vi "Distance-Speed Adaptor.vi"(4 "Sensor Data":dbl) -> (0 "Speed":dbl(slide) scale=0.0..1.0)   [LabVIEW 2019]
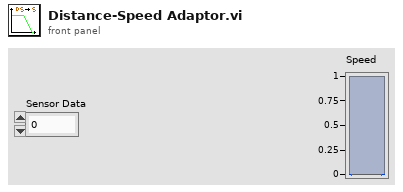
[diagram p1: front panel]
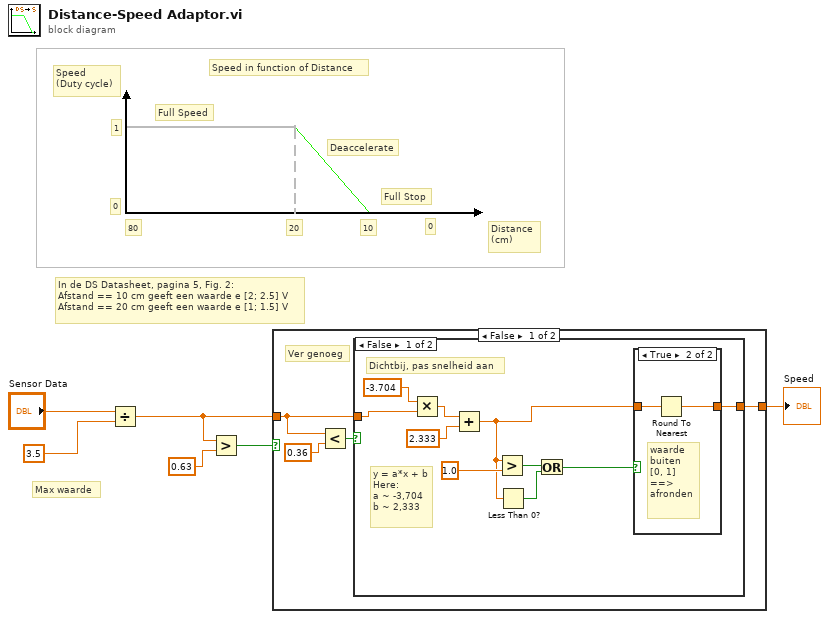
[diagram p0: block diagram]
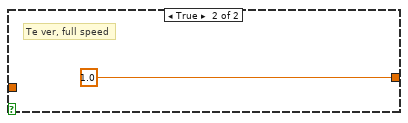
[diagram p3: hidden frame]
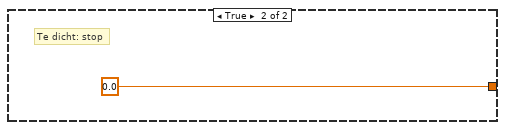
[diagram p4: hidden frame]
diagram:
  # "Max waarde"
  # "In de DS Datasheet, pagina 5, Fig. 2:\nAfstand == 10 cm geeft een waarde e [2; 2.5] V\nAfstand == 20 cm geeft een waarde e [1; 1.5] V"
  # "Speed in function of Distance"
  # "Full Stop"
  # "Deaccelerate"
  # "Full Speed"
  # "0"
  # "10"
  # "20"
  # "80"
  # "Distance\n(cm)"
  # "Speed\n(Duty cycle)"
  # "0"
  # "1"
  n1 = Divide(x="Sensor Data", y=3.5) -> (x/y=w1:dbl)
  n2 = Greater?(x=w1, y=0.63) -> (0:w3:bool)
  n3 = case shown="False" w3 {
    tunnel: [w8 0.0] -> w2
    tunnel: w1 -> [w7 _]
    frame False {
      # "Ver genoeg"
      n4 = Less?(x=w7, y=0.36) -> (x < y?=w10:bool)
      n5 = case shown="False" w10 {
        tunnel: [w12 1.0] -> w8
        tunnel: w7 -> [w19 _]
        frame False {
          # "Dichtbij, pas snelheid aan"
          # "y = a*x + b\nHere:\na ~ -3,704\nb ~ 2,333"
          n6 = Multiply(x=-3.704, y=w19) -> (x*y=w18:dbl)
          n7 = Add(x=w18, y=2.333) -> (x+y=w11:dbl)
          n8 = Greater?(x=w11, y=1.0) -> (0:w15:bool)
          n9 = Less Than 0?(x=w11) -> (x < 0?=w16:bool)
          n10 = Or(x=w15, y=w16) -> (x .or. y?=w13:bool)
          n11 = case shown="True" w13 {
            tunnel: [w21 w23] -> w12
            tunnel: w11 -> [w21 w22]
            frame False {
              # "Waarde\ne [0, 1]"
            }
            frame True {
              # "waarde\nbuiten\n[0, 1]\n==>\nafronden"
              n12 = Round To Nearest(number=w22) -> (nearest integer value=w23:dbl)
            }
          }
        }
        frame True {
          # "Te ver, full speed"
        }
      }
    }
    frame True {
      # "Te dicht: stop"
    }
  }
  "Speed" <- w2
